vi "TEST.vi"() -> ()   [LabVIEW 2016, in "Instrument UI.PPMS.lvclass"]
uses:
  Instrument UI.PPMS.lvclass
  instrument.PPMS/Typedefs/Select PPMS--Enum.ctl
  C:/Program Files (x86)/National Instruments/LabVIEW 2016/user.lib/LevyLab/Levylab Instruments/SMOs/Instrument UI/Instrument UI.lvclass
  C:/Program Files (x86)/National Instruments/LabVIEW 2016/vi.lib/JKI/JKI SMO/SMO/SMO.lvclass
  <userlib>/LevyLab/Levylab Instruments/SMOs/Instrument UI/Instrument UI.lvclass/Instrument UI.ctl
  instrument.PPMS/instrument.PPMS.lvclass
  C:/Program Files (x86)/National Instruments/LabVIEW 2016/user.lib/LevyLab/Levylab Instruments/SMOs/Instrument/Instrument.lvclass
  <userlib>/LevyLab/Levylab Instruments/SMOs/Instrument/Instrument.lvclass
  <userlib>/LevyLab/Levylab Instruments/SMOs/Instrument UI/Instrument UI.lvclass
  <vilib>/JKI/JKI SMO/SMO/SMO.lvclass
panel:
  out "Select PPMS out":T1
  in  "Select PPMS":T1
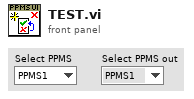
[diagram p1: front panel]
types:
  T1 = typedef "instrument.PPMS.lvclass/Select PPMS--Enum.ctl" = enum16{"PPMS1", "PPMS2", "PPMS3"}
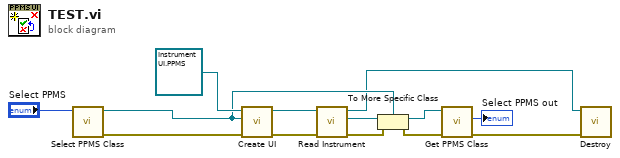
[diagram p0: block diagram]
diagram:
  n1 = call "Select PPMS Class.vi"("Select PPMS"="Select PPMS") -> ("error out"=w9:errorcluster, "instrument.PPMS out"=w8:refnum<class "instrument.PPMS.lvclass">)  [unwired: 9 in]
  n2 = call <userlib>:"Create UI.vi"("error in (no error)"=w9, "Instrument in"=w8, "Instrument UI"=refnum<class "Instrument UI.PPMS.lvclass"> refnum ("SR7220 UI.lvclass")) -> ("error out"=w11:errorcluster, "Instrument UI out"=w12:refnum<class "Instrument UI.PPMS.lvclass">)  [unwired: 7 in]
  n3 = call <userlib>:"Read Instrument.vi"("error in (no error)"=w11, "Instrument UI in"=w12) -> ("error out"=w5:errorcluster, "Instrument.lvclass"=w3:refnum<class "Instrument.lvclass">, "Instrument UI out"=w1:refnum<class "Instrument UI.PPMS.lvclass">)  [unwired: 7 in]
  n4 = To More Specific Class(target class=w8, reference=w3, error in=w5) -> (specific class reference=w7:refnum<class "instrument.PPMS.lvclass">, error out=w4:errorcluster)
  n5 = call "Get PPMS Class.vi"("error in (no error)"=w4, "instrument.PPMS"=w7) -> ("error out"=w2:errorcluster, "Select PPMS"=→"Select PPMS out":T1)  [unwired: 7 in, 1 out]
  n6 = call <vilib>:"Destroy.vi"("error in (no error)"=w2, "SMO"=w1) -> ()  [unwired: 9 in, 1 out]
